vi "2100_Read RFFE_w_Waveform.vi"(0 "Semiconductor Module Context":T2, 1 "Num_Reg_to_Read":u8=1, 5 "Pins":string[](array[string])=["CLK", "SDA"], 7 "Reg_Address_Data":T4={"Address"=81, "Data"=0} {"Address" format="%.0x"}, 9 "USID":T3 max=15, 11 "Error In":errorcluster) -> (4 "Semiconductor Module Context Out":T2, 8 "Converted Data":T5 {"Register" max=31 format="%.0x"; "Slave Address" max=15 format="%.0x"}, 15 "Error Out":errorcluster)   [LabVIEW 2013]
uses:
  <vilib>/NI_TestStand_SemiconductorModule/NI_TestStand_Semiconductor_Module.lvlibp/PinMap/General/SemiconductorModuleContext.ctl
  Controls/USID.ctl
  Controls/Reg_Address_Data.ctl
  MIPI_RFFE/Ctrls/RegReadWrite.ctl
  MIPI_RFFE/Ctrls/Configuration.ctl
  MIPI_RFFE/Ctrls/ClockDataChannels.ctl
  <vilib>/NI_TestStand_SemiconductorModule/NI_TestStand_Semiconductor_Module.lvlibp/PinMap/HSDIO/PinsToNIHSDIOSessions.vi
  <vilib>/Waveform/DWDTOps.llb/DWDT Digital Size.vi
  <instrlib>/niHSDIO/niHSDIO.llb/niHSDIO Write Named Waveform (WDT).vi
  <instrlib>/niHSDIO/niHSDIO.llb/niHSDIO Fetch Waveform (WDT).vi
  <vilib>/NI_TestStand_SemiconductorModule/NI_TestStand_Semiconductor_Module.lvlibp
panel:
  in  "Tab Control":T1(tab)
  out "Waveform Graph":digitalwaveform(graph)
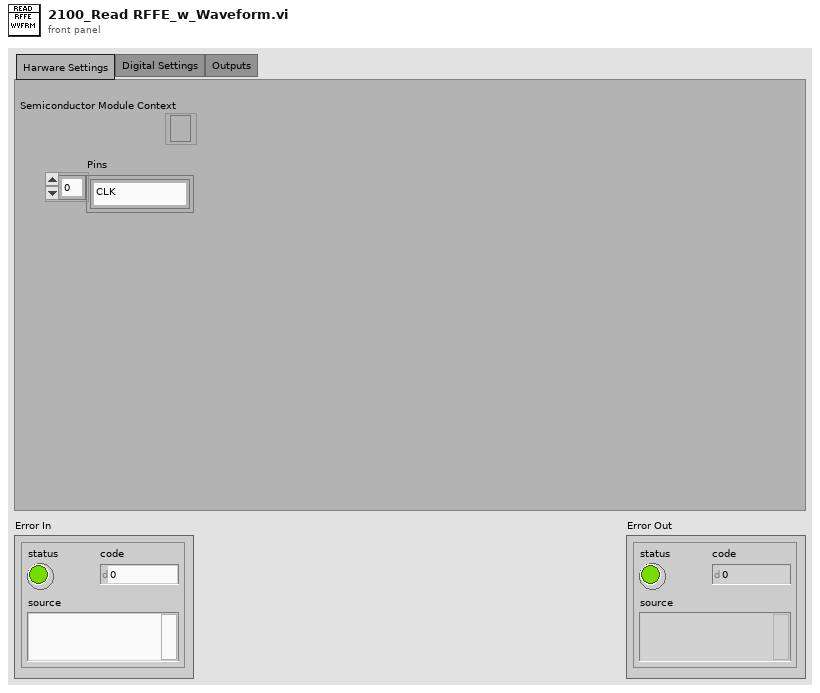
[diagram p1: front panel]
types:
  T1 = enum32{"Harware Settings", "Digital Settings", "Outputs"}
  T2 = typedef "NI_TestStand_Semiconductor_Module.lvlibp/SemiconductorModuleContext.ctl" = refnum<k7>
  T3 = typedef "USID.ctl" = u8
  T4 = typedef "Reg_Address_Data.ctl" = cluster{"Address":u8, "Data":u8}
  T5 = cluster{"Slave Address":u8, "Register":u8, "Data":u8}
  T6 = typedef "Configuration.ctl" = cluster{"Samples to Allocate":i32, "Oversample Factor":u8, "Clock Channel":T7, "Data Channel":T7}
  T7 = typedef "ClockDataChannels.ctl" = enum16{"0", "1"}
  T8 = typedef "RegReadWrite.ctl" = cluster{"Slave Address":u8, "Register":u8, "Data":u8, "SetID_Pin_State":enum16{"0", "1", "Z"}}
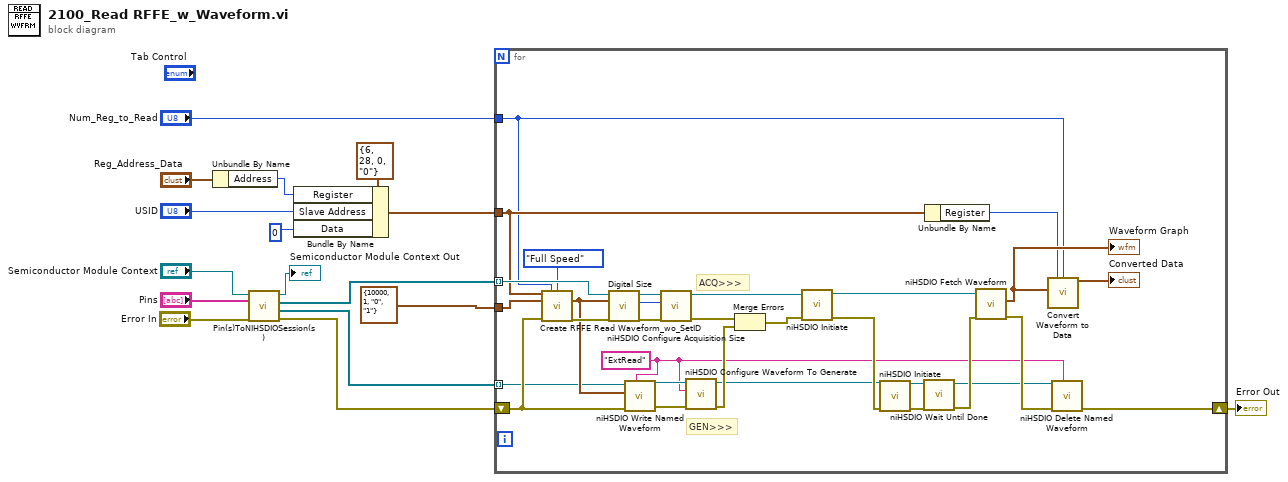
[diagram p0: block diagram]
diagram:
  n1 = Unbundle By Name("Reg_Address_Data") -> ("Address"=w4:u8)
  n2 = call-poly <vilib>:"Pin(s)ToNIHSDIOSession(s).vi"("error in (no error)"="Error In", "Pins"="Pins", "Semiconductor Module Context"="Semiconductor Module Context") -> ("error out"=w14:errorcluster, "Generation Sessions"=w15:refnum<k15>[], "Acquisition Sessions"=w16:refnum<k15>[], "Semiconductor Module Context Out"=→"Semiconductor Module Context Out":T2)  [unwired: 3 in, 2 out]
  n3 = Bundle By Name(cluster=T8 {"Slave Address"=6, "Register"=28, "Data"=0, "SetID_Pin_State"=enum."0"} ("Data"), "Register"=w4, "Slave Address"="USID", "Data"=u8 0) -> (w9:T8)
  n4 = for {
    tunnel: w16 -> [w39] mode=indexing
    tunnel: w15 -> [w22] mode=indexing
    tunnel: w9 -> [w24]
    tunnel: T6 {"Samples to Allocate"=10000, "Oversample Factor"=1, "Clock Channel"=enum."0", "Data Channel"=enum."1"} ("Configuratation") -> [w37]
    shift-right: [w17] -> w2
    shift-left: w14 -> [w23]
    tunnel: "Num_Reg_to_Read" -> [w18]
    w26 = "ExtRead" ("waveform name (default:\"\")")
    # "GEN>>>"
    # "ACQ>>>"
    n5 = call "Create RFFE Read Waveform_wo_SetID.vi"("Data"=w24, "Ext_Read_Num_Reg"=w18, "Readback Speed"=enum16{"Full Speed", "Half Speed"}."Full Speed", "Configuratation"=w37, "error in (no error)"=w23) -> ("Waveform Graph"=w25:digitalwaveform, "error out"=w40:errorcluster)  [unwired: 9 in]
    n6 = call-poly <vilib>:"Digital Size.vi"("error in (no error)"=w40, "digital waveform in"=w25) -> ("error out"=w41:errorcluster, "number of samples"=w42:i32)  [unwired: 6 in, 2 out]
    n7 = call-poly <instrlib>:"niHSDIO Write Named Waveform.vi"("waveform name (default:\"\")"=w26, "error in (no error)"=w23, "data"=w25, "instrument handle"=w22) -> ("error out"=w32:errorcluster, "instrument handle out"=w30:refnum<k15>)  [unwired: 6 in]
    n8 = call <instrlib>:"niHSDIO Configure Acquisition Size.vi"("error in (no error)"=w41, "samples per record (1000 samples)"=w42, "instrument handle"=w39) -> ("error out"=w38:errorcluster, "instrument handle out"=w43:refnum<k15>)  [unwired: 7 in]
    n9 = call <instrlib>:"niHSDIO Configure Waveform To Generate.vi"("error in (no error)"=w32, "waveform name"=w26, "instrument handle"=w30) -> ("error out"=w31:errorcluster, "instrument handle out"=w29:refnum<k15>)  [unwired: 7 in]
    n10 = Merge Errors(w38, w31) -> (w44:errorcluster)
    n11 = call <instrlib>:"niHSDIO Initiate.vi"("error in (no error)"=w44, "instrument handle"=w43) -> ("error out"=w46:errorcluster, "instrument handle out"=w33:refnum<k15>)  [unwired: 8 in]
    n12 = call <instrlib>:"niHSDIO Initiate.vi"("error in (no error)"=w46, "instrument handle"=w29) -> ("error out"=w45:errorcluster, "instrument handle out"=w34:refnum<k15>)  [unwired: 8 in]
    n13 = call <instrlib>:"niHSDIO Wait Until Done.vi"("error in (no error)"=w45, "instrument handle"=w34) -> ("error out"=w36:errorcluster, "instrument handle out"=w27:refnum<k15>)  [unwired: 8 in]
    n14 = Unbundle By Name(w24) -> ("Register"=w19:u8)
    n15 = call-poly <instrlib>:"niHSDIO Fetch Waveform.vi"("error in (no error)"=w36, "instrument handle"=w33) -> ("error out"=w28:errorcluster, "data"=w21:digitalwaveform)  [unwired: 6 in, 2 out]
    "Waveform Graph" <- w21
    n16 = call "Convert Waveform to Data.vi"("Waveform Graph"=w21, "Register"=w19, "Ext_Read_Num_Reg"=w18) -> ("Converted Data"=→"Converted Data":T5)  [unwired: 10 in, 2 out]
    n17 = call <instrlib>:"niHSDIO Delete Named Waveform.vi"("waveform name (default:\"\")"=w26, "error in (no error)"=w28, "instrument handle"=w27) -> ("error out"=w17:errorcluster)  [unwired: 7 in, 1 out]
  }
  "Error Out" <- w2
